vi "火球和小怪物.vi"() -> ()   [LabVIEW 2018]
panel:
  out "布尔":bool
  in  "滑动杆":dbl(slide) scale=0.0..10.0
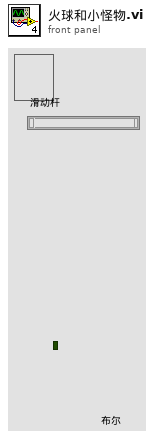
[diagram p1: front panel]
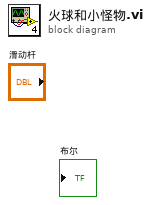
[diagram p0: block diagram]
diagram:
